vi "Initialise IO.vi"(8 "error in (no error)":errorcluster) -> (0 "error out":errorcluster, 3 "IO":T1)   [LabVIEW 2021, in "Test Sequencer Support.lvlib"]
uses:
  Test Sequencer Support.lvlib
  IO Type.ctl
  <vilib>/TSA/Event Log/Event_TextLog/Event_TextLog.lvclass
  C:/Program Files (x86)/National Instruments/LabVIEW 2021/vi.lib/TSA/Event Log/abs_EventLog/abs_EventLog.lvclass
  Blackboard/Blackboard.lvclass
  <vilib>/TSA/Abstract Data Classes/Abs_Types/Boolean/Abs_Boolean.lvclass
  <vilib>/TSA/Abstract Data Classes/Abs_Types/Waveform/Abs_Waveform.lvclass
  <vilib>/TSA/Abstract Data Classes/Abs_Types/Double Float/Abs_Double Float.lvclass
  C:/Program Files (x86)/National Instruments/LabVIEW 2021/vi.lib/TSA/Abstract Data Classes/Abs_Types/Numeric/Abs_Numeric.lvclass
  <vilib>/TSA/Event Log/abs_EventLog/Support/Severity Code.ctl
  Blackboard/Blackboard.lvclass/Blackboard.ctl
  <vilib>/TSA/Abstract Data Classes/Abs_Types/Numeric/Abs_Numeric.lvclass/Abs_Numeric.ctl
  <vilib>/TSA/Event Log/abs_EventLog/abs_EventLog.lvclass/abs_EventLog.ctl
  Blackboard/Get Value Type/Get Boolean.vi
  Blackboard/Get Value Type/Get Waveform.vi
  Blackboard/Get Value Type/Get DBL.vi
  <vilib>/TSA/Abstract Data Classes/Abs_Types/Numeric/Properties/Write Units.vi
  <vilib>/TSA/Event Log/abs_EventLog/Properties/Write Severity Code.vi
  Blackboard/Support/Index Group.vi
  Blackboard/Support/Index Tags.vi
  <vilib>/TSA/Omni-Bus/Local Bus/Support/Bool/Local Bus_Boolean.lvclass
  C:/Program Files (x86)/National Instruments/LabVIEW 2021/vi.lib/TSA/Abstract Data Classes/Abs_Types/Value/Abs_Value.lvclass
  <vilib>/TSA/Omni-Bus/Local Bus/Support/WFM/Local Bus_Waveform.lvclass
  <vilib>/TSA/Omni-Bus/Local Bus/Support/DBL/Local Bus_DBL.lvclass
  <vilib>/TSA/Omni-Bus/Local Bus/Support/Initialise DVR's.vi
  <vilib>/TSA/Abstract Data Classes/Abs_Types/Value/Abs_Value.lvclass
  <vilib>/TSA/Abstract Data Classes/Abs_Types/Type/Abs_Type.lvclass
  <vilib>/TSA/Omni-Bus/Local Bus/Support/SGL/Local Bus_SGL.lvclass
  <vilib>/TSA/Omni-Bus/Local Bus/Support/EXT/Local Bus_EXT.lvclass
  <vilib>/TSA/Omni-Bus/Local Bus/Support/STR/Local Bus_String.lvclass
  <vilib>/TSA/Omni-Bus/Local Bus/Support/Variant/Local Bus_Variant.lvclass
  <vilib>/TSA/Omni-Bus/Local Bus/Support/Time/Local Bus_Time.lvclass
  <vilib>/TSA/Omni-Bus/Local Bus/Support/U8/Local Bus_U8.lvclass
  <vilib>/TSA/Omni-Bus/Local Bus/Support/U16/Local Bus_U16.lvclass
  <vilib>/TSA/Omni-Bus/Local Bus/Support/U32/Local Bus_U32.lvclass
  <vilib>/TSA/Omni-Bus/Local Bus/Support/U64/Local Bus_U64.lvclass
  <vilib>/TSA/Omni-Bus/Local Bus/Support/I8/Local Bus_I8.lvclass
  <vilib>/TSA/Omni-Bus/Local Bus/Support/I16/Local Bus_I16.lvclass
  <vilib>/TSA/Omni-Bus/Local Bus/Support/I32/Local Bus_I32.lvclass
  <vilib>/TSA/Omni-Bus/Local Bus/Support/I64/Local Bus_I64.lvclass
  <vilib>/TSA/Omni-Bus/Local Bus/Support/CSGL/Local Bus_CSGL.lvclass
  <vilib>/TSA/Omni-Bus/Local Bus/Support/CDBL/Local Bus_CDBL.lvclass
  <vilib>/TSA/Omni-Bus/Local Bus/Support/CEXT/Local Bus_CEXT.lvclass
  <vilib>/TSA/Omni-Bus/Local Bus/Support/Type/Local Bus_Type.lvclass
  <vilib>/TSA/Event Log/abs_EventLog/abs_EventLog.lvclass
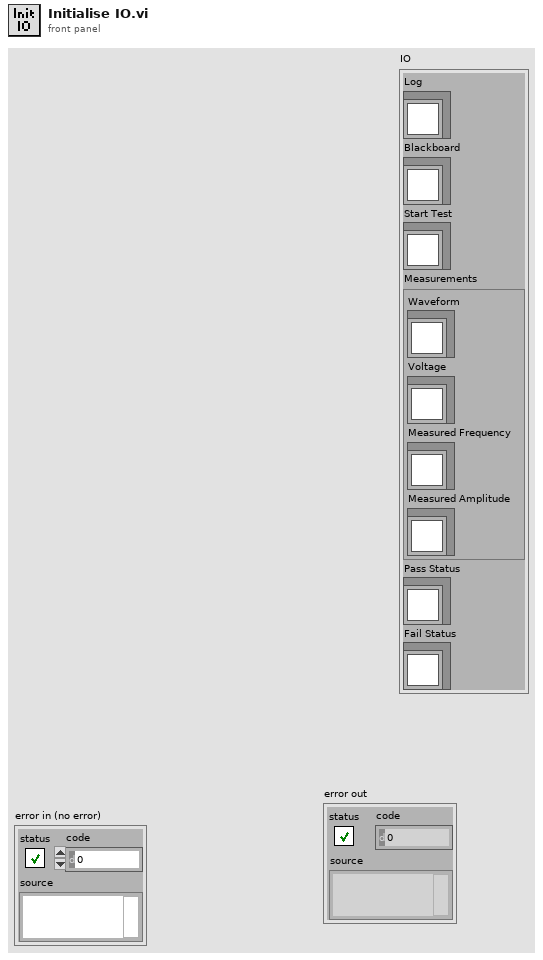
[diagram p1: front panel]
types:
  T1 = typedef "Test Sequencer Support.lvlib/IO Type.ctl" = cluster{"Log":refnum<class "Event_TextLog.lvclass">, "Blackboard":refnum<class "Blackboard.lvclass">, "Start Test":refnum<class "Abs_Boolean.lvclass">, "Measurements":cluster{"Waveform":refnum<class "Abs_Waveform.lvclass">, "Voltage":refnum<class "Abs_Double Float.lvclass">, "Measured Frequency":refnum<class "Abs_Double Float.lvclass">, "Measured Amplitude":refnum<class "Abs_Double Float.lvclass">}, "Pass Status":refnum<class "Abs_Boolean.lvclass">, "Fail Status":refnum<class "Abs_Boolean.lvclass">}
  T2 = typedef "abs_EventLog.lvclass/Severity Code.ctl" = enum16{"emergency", "alert", "critical", "error", "warning", "notice", "info", "debug"}
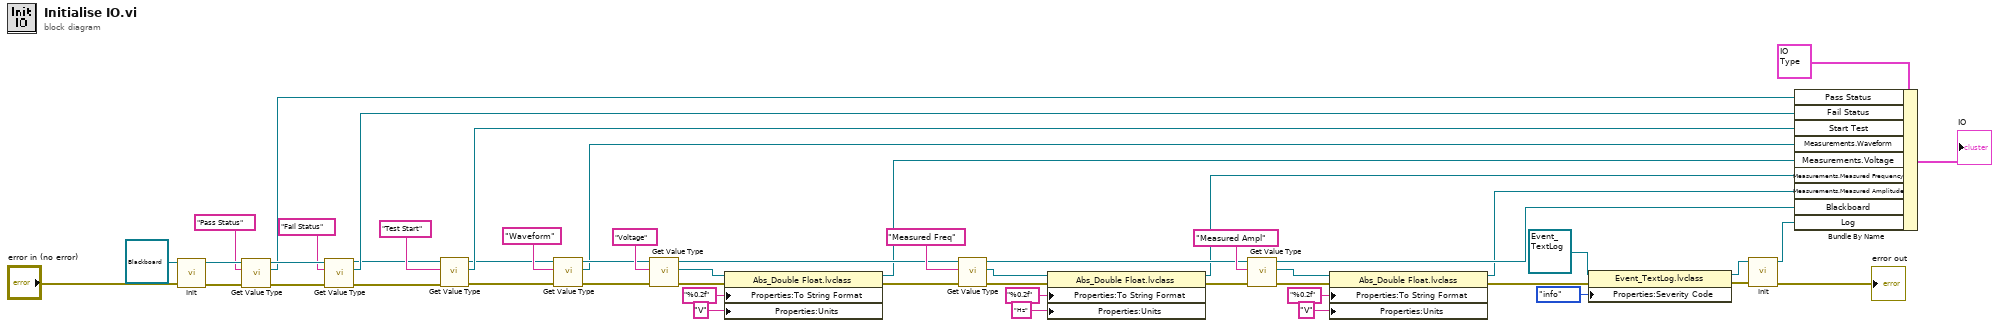
[diagram p0: block diagram]
diagram:
  n1 = call-dynamic "Init.vi"("error in (no error)"="error in (no error)", "bt_Blackboard in"=refnum<class "Blackboard.lvclass"> refnum) -> ("error out"=w30:errorcluster, "bt_Blackboard out"=w29:refnum<class "Blackboard.lvclass">)  [unwired: 8 in]
  n2 = call-poly "Get Value Type.vi"("error in (no error)"=w30, "Tag"="Pass Status", "Blackboard in"=w29) -> ("error out"=w27:errorcluster, "Value"=w26:refnum<class "Abs_Boolean.lvclass">, "Blackboard out"=w28:refnum<class "Blackboard.lvclass">)  [unwired: 5 in, 1 out]
  n3 = call-poly "Get Value Type.vi"("error in (no error)"=w27, "Tag"="Fail Status", "Blackboard in"=w28) -> ("error out"=w32:errorcluster, "Value"=w33:refnum<class "Abs_Boolean.lvclass">, "Blackboard out"=w31:refnum<class "Blackboard.lvclass">)  [unwired: 5 in, 1 out]
  n4 = call-poly "Get Value Type.vi"("error in (no error)"=w32, "Tag"="Test Start", "Blackboard in"=w31) -> ("error out"=w39:errorcluster, "Value"=w41:refnum<class "Abs_Boolean.lvclass">, "Blackboard out"=w38:refnum<class "Blackboard.lvclass">)  [unwired: 5 in, 1 out]
  n5 = call-poly "Get Value Type.vi"("error in (no error)"=w39, "Tag"="Waveform", "Blackboard in"=w38) -> ("error out"=w35:errorcluster, "Value"=w34:refnum<class "Abs_Waveform.lvclass">, "Blackboard out"=w36:refnum<class "Blackboard.lvclass">)  [unwired: 5 in, 1 out]
  n6 = call-poly "Get Value Type.vi"("error in (no error)"=w35, "Tag"="Voltage", "Blackboard in"=w36) -> ("error out"=w18:errorcluster, "Value"=w17:refnum<class "Abs_Double Float.lvclass">, "Blackboard out"=w22:refnum<class "Blackboard.lvclass">)  [unwired: 5 in, 1 out]
  n7 = property class="Abs_Double Float.lvclass"(reference=w17, error in=w18, "Properties:To String Format"="%0.2f" ("To String Format"), "Properties:Units"="V" ("Units")) -> (reference out=w14:refnum<class "Abs_Double Float.lvclass">, error out=w13:errorcluster)
  n8 = call-poly "Get Value Type.vi"("error in (no error)"=w13, "Tag"="Measured Freq", "Blackboard in"=w22) -> ("error out"=w9:errorcluster, "Value"=w7:refnum<class "Abs_Double Float.lvclass">, "Blackboard out"=w20:refnum<class "Blackboard.lvclass">)  [unwired: 5 in, 1 out]
  n9 = property class="Abs_Double Float.lvclass"(reference=w7, error in=w9, "Properties:To String Format"="%0.2f" ("To String Format"), "Properties:Units"="Hz" ("Units")) -> (reference out=w8:refnum<class "Abs_Double Float.lvclass">, error out=w10:errorcluster)
  n10 = call-poly "Get Value Type.vi"("error in (no error)"=w10, "Tag"="Measured Ampl", "Blackboard in"=w20) -> ("error out"=w4:errorcluster, "Value"=w1:refnum<class "Abs_Double Float.lvclass">, "Blackboard out"=w19:refnum<class "Blackboard.lvclass">)  [unwired: 5 in, 1 out]
  n11 = property class="Abs_Double Float.lvclass"(reference=w1, error in=w4, "Properties:To String Format"="%0.2f" ("To String Format"), "Properties:Units"="V" ("Units")) -> (reference out=w2:refnum<class "Abs_Double Float.lvclass">, error out=w3:errorcluster)
  n12 = property class="Event_TextLog.lvclass"(reference=refnum<class "Event_TextLog.lvclass"> refnum ("Event_TextLog in"), error in=w3, "Properties:Severity Code"=Severity_Code."info" ("Severity Code")) -> (reference out=w43:refnum<class "Event_TextLog.lvclass">, error out=w44:errorcluster)
  n13 = call-dynamic "Init.vi"("error in (no error)"=w44, "Event_TextLog in"=w43) -> ("error out"=→"error out":errorcluster, "Event_TextLog out"=w48:refnum<class "Event_TextLog.lvclass">)  [unwired: 8 in]
  n14 = Bundle By Name(cluster=T1 {"Log"=refnum, "Blackboard"=refnum, "Start Test"=refnum, "Measurements"={"Waveform"=refnum, "Voltage"=refnum, "Measured Frequency"=refnum, "Measured Amplitude"=refnum}, "Pass Status"=refnum, "Fail Status"=refnum} ("IO"), "Pass Status"=w26, "Fail Status"=w33, "Start Test"=w41, "Measurements.Waveform"=w34, "Measurements.Voltage"=w14, "Measurements.Measured Frequency"=w8, "Measurements.Measured Amplitude"=w2, "Blackboard"=w19, "Log"=w48) -> (→"IO":T1)
